vi "climb mode.vi"(4 "i":i32=1508, 6 "Joystick 2":T1, 7 "Arm Angle":dbl=0.38043151000000003, 8 "engage climb":bool, 9 "Button 1":bool, 10 "Slide":dbl(slide)=1.0 scale=0.0..1.0, 11 "Joystick 1 Axes":T2={"Axis 1 (x)"=0.047244094488188976, "Axis 2 (y)"=-0.047244094488188976, "Axis 3 (throttle)"=-1.0, "Axis 4"=0.0, "Axis 5"=0.0, "Axis 6"=0.0}) -> ()   [LabVIEW 2012]
uses:
  <vilib>/Rock Robotics/WPI/Solenoid/WPI_SolenoidValue.ctl
  <vilib>/Rock Robotics/WPI/Joystick/WPI_JoystickGetSetRefNum.vi
  <vilib>/Rock Robotics/WPI/Solenoid/WPI_SolenoidSetEnum.vi
panel:
  out "Arm Motor Output":dbl
  out "Down Range":dbl=0.6
  out "Up Range":dbl=4.1
  out "right f":i32=11868
  out "left f":i32=11868
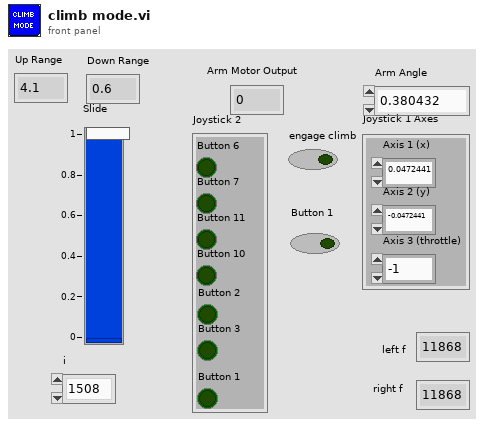
[diagram p1: front panel]
types:
  T1 = cluster{"Button 6":bool, "Button 7":bool, "Button 11":bool, "Button 10":bool, "Button 2":bool, "Button 3":bool, "Button 1":bool}
  T2 = cluster{"Axis 1 (x)":dbl, "Axis 2 (y)":dbl, "Axis 3 (throttle)":dbl, "Axis 4":dbl, "Axis 5":dbl, "Axis 6":dbl}
  T3 = typedef "WPI_SolenoidValue.ctl" = enum16{"Off", "On", "Forward", "Reverse"}
  T4 = typedef "WPI_JoystickDevRef.ctl" = cluster{"Device":T5}
  T5 = typedef "WPI_JoystickDeviceEnum.ctl" = enum16{"USB 1", "USB 2", "USB 3", "USB 4", "Kinect 1", "Kinect 2"}
  T6 = typedef "WPI_JoystickButtonState.ctl" = cluster{"Button 1":bool, "Button 2":bool, "Button 3":bool, "Button 4":bool, "Button 5":bool, "Button 6":bool, "Button 7":bool, "Button 8":bool, "Button 9":bool, "Button 10":bool, "Button 11":bool, "Button 12":bool}
  T7 = typedef "WPI_MotorControlDeviceRef.ctl" = cluster{"DeviceStatus":errorcluster, "Type":enum16{"PWM", "CAN"}, "PWM":cluster{"Digital Module":T8, "PWM Channel":T9, "DeadBand":T10}, "CAN":cluster{"Device Number":u8, "Control Mode":T11, "Semaphore":T12, "Max Vout":dbl}, "Invert":bool, "TransformRef":T13, "InvTransformRef":T13}
  T8 = typedef "FPGA_TypedefDigitalModule.ctl" = enum16{"Digital Module 1", "Digital Module 2"}
  T9 = typedef "FPGA_DIOPWMChannel.ctl" = enum8{"PWM 1", "PWM 2", "PWM 3", "PWM 4", "PWM 5", "PWM 6", "PWM 7", "PWM 8", "PWM 9", "PWM 10", "Invalid"}
  T10 = typedef "WPI_PWMDeadband.ctl" = cluster{"Name":string, "maxPositivePwm":i32, "minPositivePwm":i32, "centerPwm":i32, "maxNegativePwm":i32, "minNegativePwm":i32, "angularRange":u16}
  T11 = typedef "WPI_CANJaguar_ControlMode.ctl" = enum8{"Percent VBus", "Current", "Speed", "Position", "Voltage"}
  T12 = typedef "Semaphore RefNum" = refnum<k1>
  T13 = typedef "WPI_PWMTransform_ConPane.ctl" = refnum<vi>
  T14 = typedef "WPI_SolenoidDevRef.ctl" = cluster{"DevStatus":errorcluster, "Solenoid Module":T15, "Forward Solenoid Channel":T16, "Reverse Solenoid Channel":T16}
  T15 = typedef "FPGA_TypedefSolenoidModule.ctl" = enum16{"Solenoid Module 1", "Solenoid Module 2"}
  T16 = typedef "WPI_SolenoidChannel.ctl" = enum8{"Solenoid 1", "Solenoid 2", "Solenoid 3", "Solenoid 4", "Solenoid 5", "Solenoid 6", "Solenoid 7", "Solenoid 8", "Invalid"}
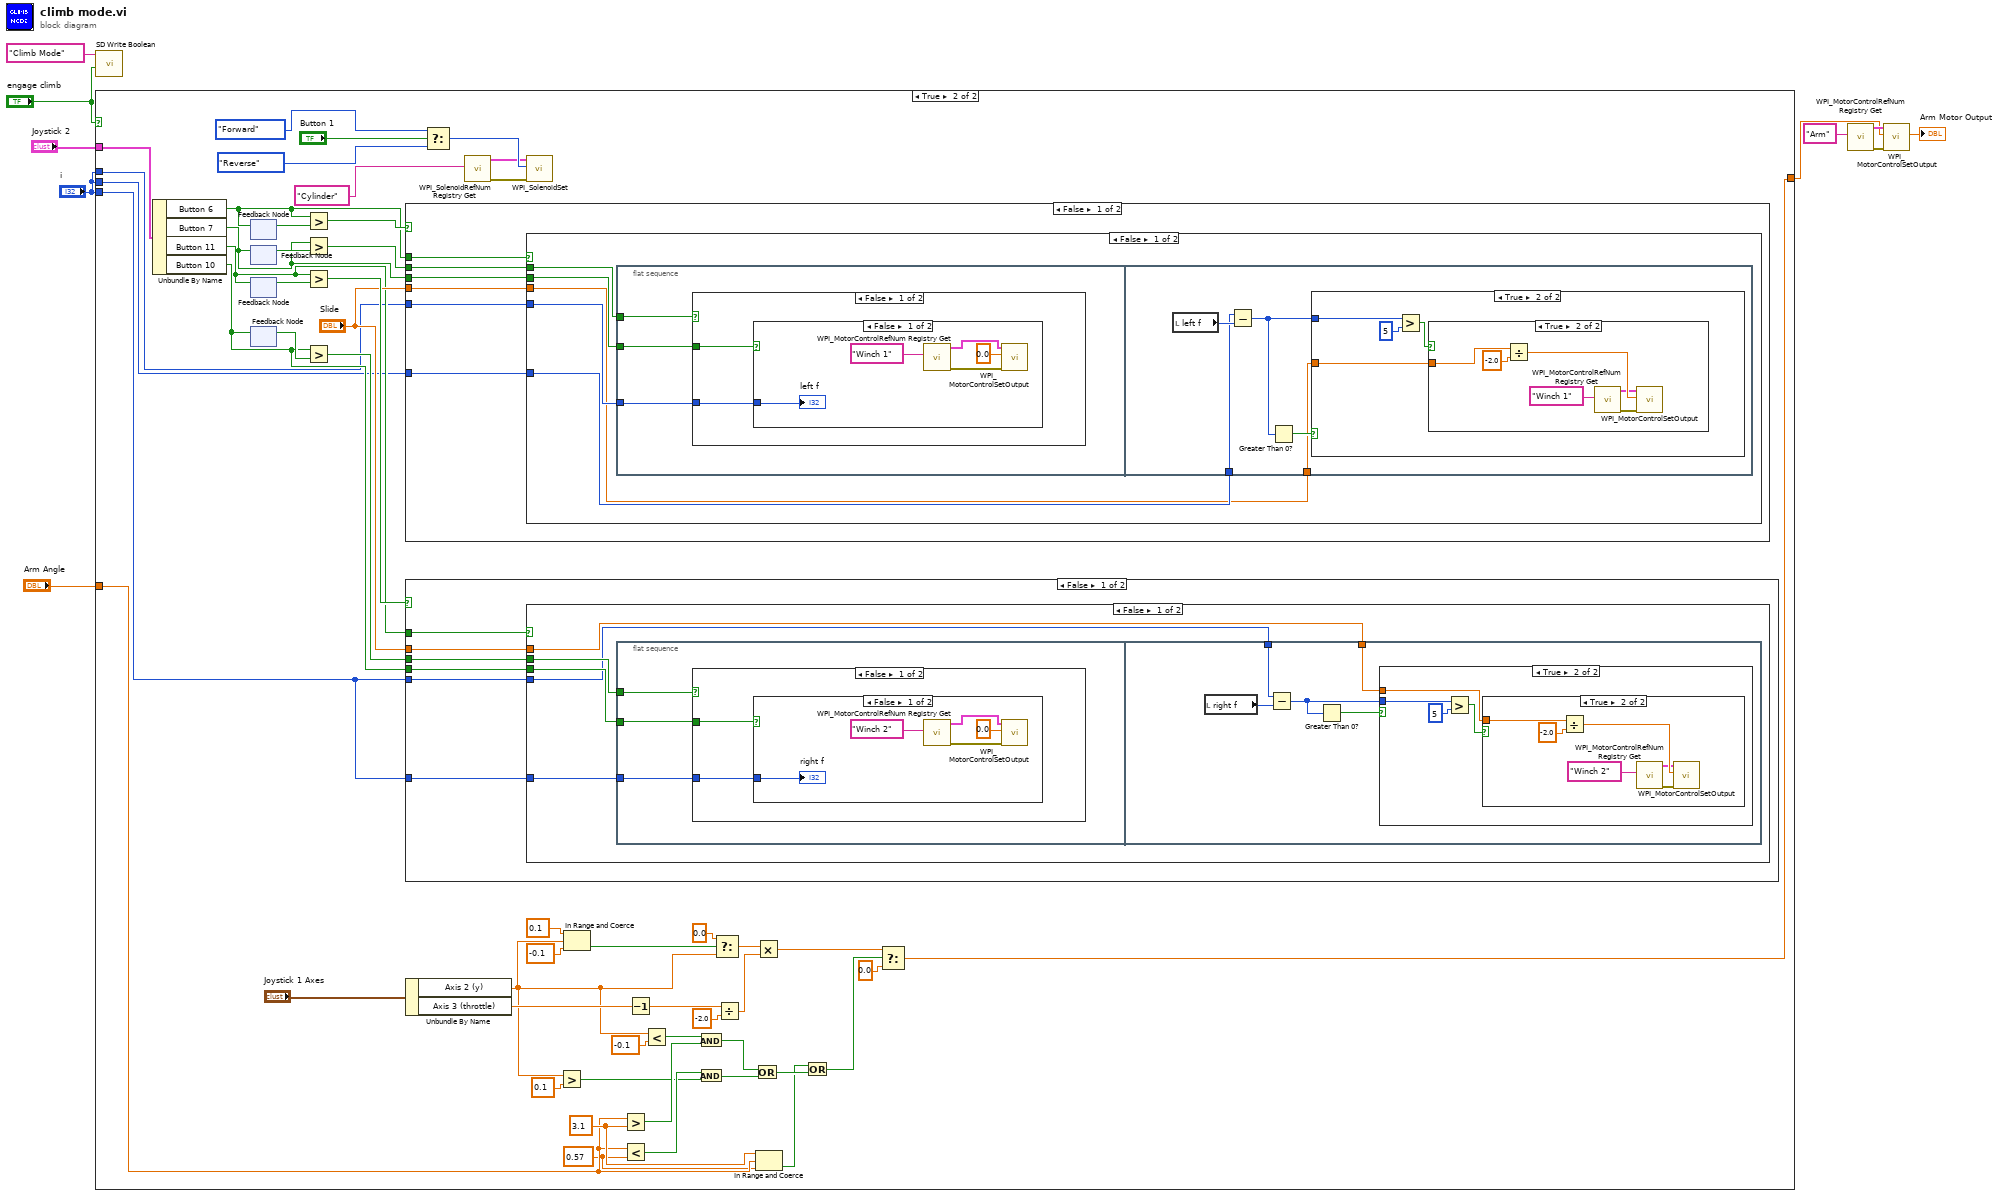
[diagram p0: block diagram]
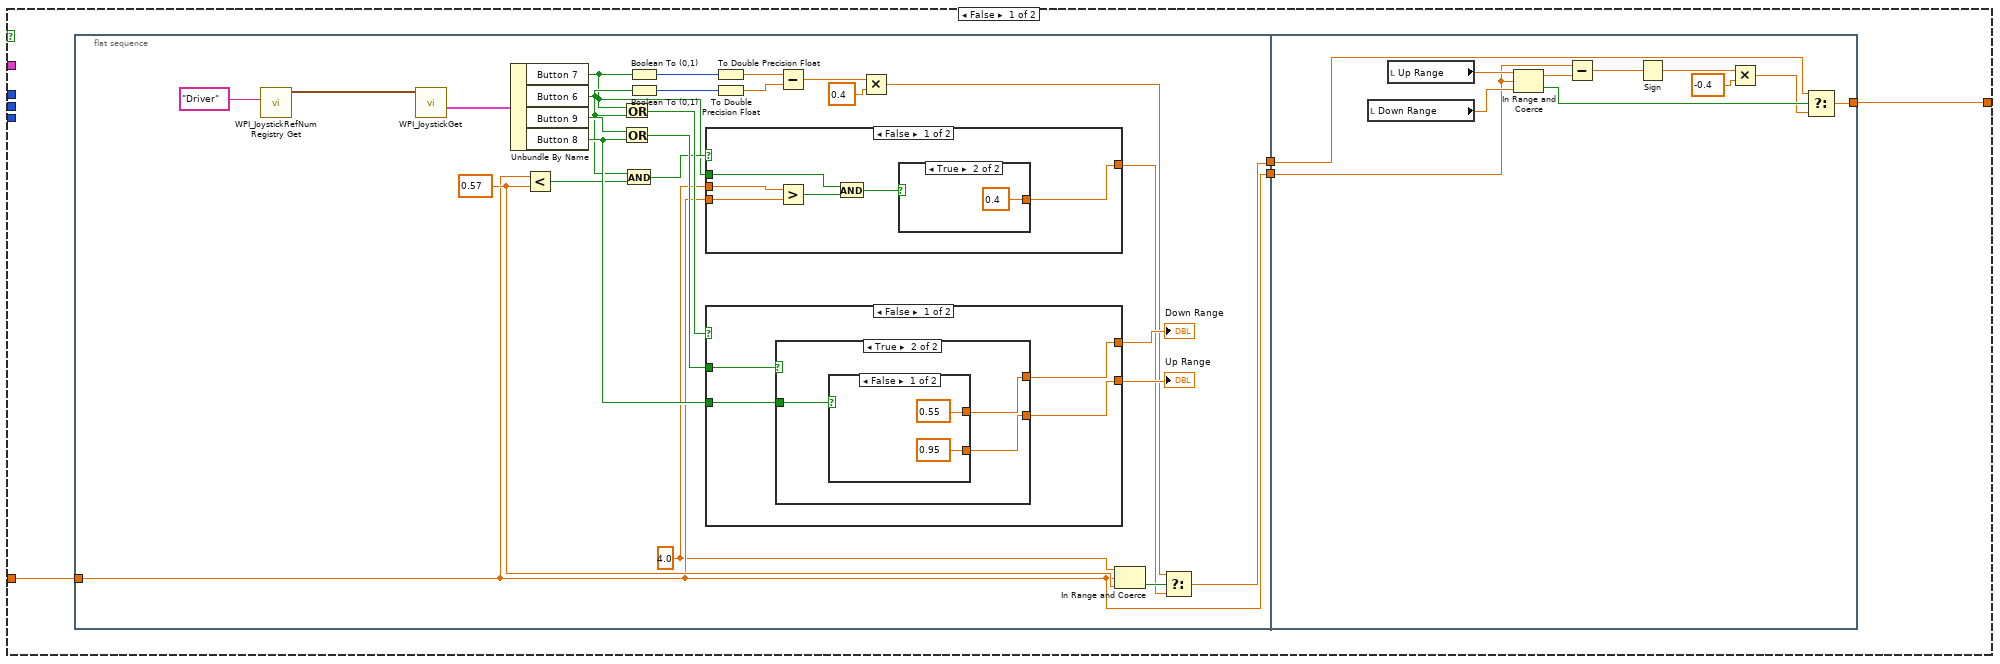
[diagram p2: hidden frame]
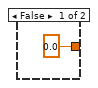
[diagram p3: hidden frame]
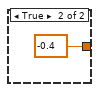
[diagram p4: hidden frame]
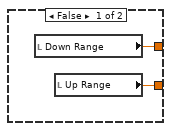
[diagram p5: hidden frame]
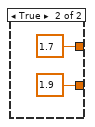
[diagram p6: hidden frame]
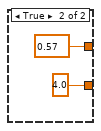
[diagram p7: hidden frame]
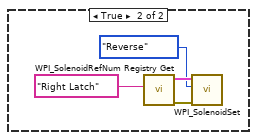
[diagram p8: hidden frame]
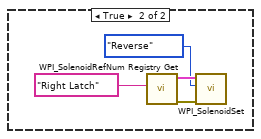
[diagram p9: hidden frame]
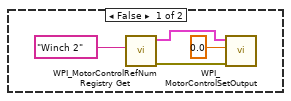
[diagram p10: hidden frame]
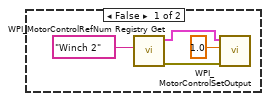
[diagram p11: hidden frame]
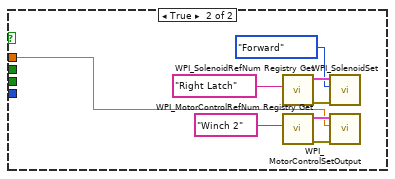
[diagram p12: hidden frame]
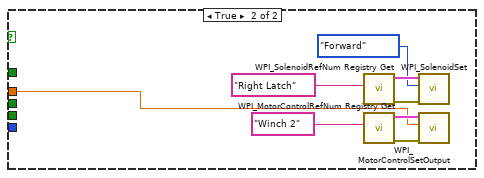
[diagram p13: hidden frame]
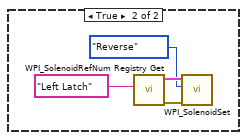
[diagram p14: hidden frame]
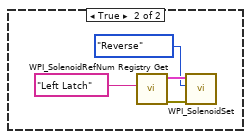
[diagram p15: hidden frame]
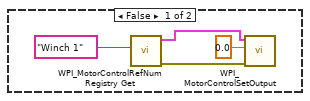
[diagram p16: hidden frame]
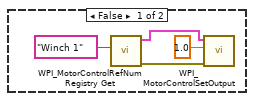
[diagram p17: hidden frame]
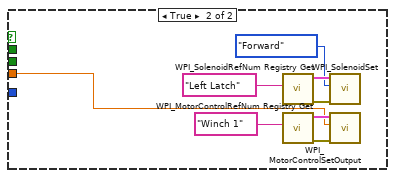
[diagram p18: hidden frame]
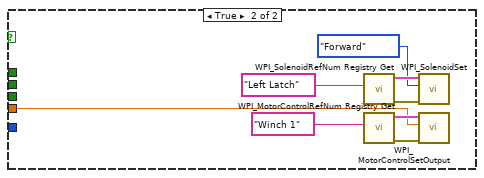
[diagram p19: hidden frame]
diagram:
  n1 = call <vilib>:"SD Write Boolean.vi"("Boolean"="engage climb", "Name"="Climb Mode") -> ()  [unwired: 8 in, 2 out]
  n2 = case shown="True" "engage climb" {
    tunnel: "Joystick 2" -> [_ w119]
    tunnel: "i" -> [_ w105]
    tunnel: "i" -> [_ w104]
    tunnel: "i" -> [_ w103]
    tunnel: "Arm Angle" -> [w14 w86]
    tunnel: [w11 w92] -> w2
    frame False {
      n3 = flat-sequence {
        tunnel: w14 -> [w16]
        tunnel: [w23] -> w13
        tunnel: [w16] -> w12
        tunnel: w13 -> [w66]
        tunnel: w12 -> [w71]
        tunnel: [w65] -> w11
        frame #0 {
          w22 = 0.57 ("lower limit")
          w15 = 4.0 ("upper limit")
          n4 = call <vilib>:"WPI_JoystickRefNum Registry Get.vi"("refnum name"="Driver") -> ("JoystickDevRef"=w40:T4)  [unwired: 9 in, 1 out]
          n5 = call <vilib>:"WPI_JoystickGet.vi"("JoystickDevRef"=w40) -> ("Buttons"=w38:T6)  [unwired: 4 in, 2 out]
          n6 = Unbundle By Name(w38) -> ("Button 7"=w17:bool, "Button 6"=w18:bool, "Button 9"=w29:bool, "Button 8"=w25:bool)
          n7 = Less?(x=w16, y=w22) -> (x < y?=w20:bool)
          n8 = Or(x=w17, y=w18) -> (x .or. y?=w28:bool)
          n9 = Or(x=w29, y=w25) -> (x .or. y?=w30:bool)
          n10 = And(x=w18, y=w20) -> (x .and. y?=w19:bool)
          n11 = Boolean To (0,1)(Boolean=w17) -> (0, 1=w37:i16)
          n12 = Boolean To (0,1)(Boolean=w18) -> (0, 1=w36:i16)
          n13 = case shown="False" w19 {
            tunnel: [w41 -0.4 ("t")] -> w21
            tunnel: w17 -> [w45 _]
            tunnel: w16 -> [w43 _]
            tunnel: w15 -> [w42 _]
            frame False {
              n14 = Greater?(x=w42, y=w43) -> (0:w44:bool)
              n15 = And(x=w45, y=w44) -> (x .and. y?=w46:bool)
              n16 = case shown="True" w46 {
                tunnel: [0.0 0.4] -> w41
                frame False {
                }
                frame True {
                }
              }
            }
            frame True {
            }
          }
          n17 = case shown="False" w28 {
            tunnel: w30 -> [w53 _]
            tunnel: [w52 4.0] -> w27
            tunnel: [w51 0.57] -> w26
            tunnel: w25 -> [w50 _]
            frame False {
              n18 = case shown="True" w53 {
                tunnel: [w55 w56] -> w52
                tunnel: [w54 w57] -> w51
                tunnel: w50 -> [_ w58]
                frame False {
                  n19 = local read "Down Range"() -> (w54:dbl)
                  n20 = local read "Up Range"() -> (w55:dbl)
                }
                frame True {
                  n21 = case shown="False" w58 {
                    tunnel: [0.55 1.7] -> w57
                    tunnel: [0.95 1.9] -> w56
                    frame False {
                    }
                    frame True {
                    }
                  }
                }
              }
            }
            frame True {
            }
          }
          "Up Range" <- w27
          "Down Range" <- w26
          n22 = To Double Precision Float(number=w37) -> (double precision float=w35:dbl)
          n23 = To Double Precision Float(number=w36) -> (double precision float=w34:dbl)
          n24 = Subtract(x=w35, y=w34) -> (x-y=w32:dbl)
          n25 = Multiply(x=w32, y=0.4) -> (x*y=w24:dbl)
          n26 = In Range and Coerce(upper limit=w15, x=w16, lower limit=w22) -> (In Range?=w31:bool)  [unwired: 1 out]
          n27 = Select(t=w24, s=w31, f=w21) -> (s? t:f=w23:dbl)
        }
        frame #1 {
          n28 = local read "Down Range"() -> (w75:dbl)
          n29 = local read "Up Range"() -> (w74:dbl)
          n30 = In Range and Coerce(upper limit=w74, x=w71, lower limit=w75) -> (coerced(x)=w72:dbl, In Range?=w73:bool)
          n31 = Subtract(x=w71, y=w72) -> (x-y=w70:dbl)
          n32 = Sign(1:w70) -> (0:w69:dbl)
          n33 = Multiply(x=w69, y=-0.4) -> (x*y=w67:dbl)
          n34 = Select(t=w66, s=w73, f=w67) -> (s? t:f=w65:dbl)
        }
      }
    }
    frame True {
      w85 = 0.57 ("lower limit")
      w87 = 3.1 ("upper limit")
      n35 = Unbundle By Name(w119) -> ("Button 6"=w109:bool, "Button 7"=w108:bool, "Button 11"=w107:bool, "Button 10"=w106:bool)
      n36 = feedback-in #1(w109) -> ()
      n37 = feedback #1() -> (w118:bool)  [unwired: 1 in]
      n38 = feedback #2() -> (w117:bool)  [unwired: 1 in]
      n39 = feedback-in #2(w108) -> ()
      n40 = feedback #3() -> (w114:bool)  [unwired: 1 in]
      n41 = feedback-in #3(w107) -> ()
      n42 = feedback #4() -> (w113:bool)  [unwired: 1 in]
      n43 = feedback-in #4(w106) -> ()
      n44 = Greater?(x=w109, y=w118) -> (0:w116:bool)
      n45 = Greater?(x=w108, y=w117) -> (0:w115:bool)
      n46 = Greater?(x=w107, y=w114) -> (0:w112:bool)
      n47 = Greater?(x=w106, y=w113) -> (0:w111:bool)
      n48 = case shown="False" w116 {
        tunnel: "Slide" -> [w200 w256]
        tunnel: w109 -> [w201 _]
        tunnel: w115 -> [w199 _]
        tunnel: w108 -> [w198 _]
        tunnel: w105 -> [w197 _]
        tunnel: w104 -> [w196 _]
        frame False {
          n49 = case shown="False" w201 {
            tunnel: w200 -> [w202 w252]
            tunnel: w198 -> [w206 _]
            tunnel: w199 -> [w205 _]
            tunnel: w197 -> [w204 _]
            tunnel: w196 -> [w203 _]
            frame False {
              n50 = flat-sequence {
                tunnel: w206 -> [w209]
                tunnel: w205 -> [w208]
                tunnel: w204 -> [w207]
                tunnel: w203 -> [w226]
                tunnel: w202 -> [w225]
                frame #0 {
                  n51 = case shown="False" w208 {
                    tunnel: w209 -> [w211 _]
                    tunnel: w207 -> [w210 _]
                    frame False {
                      n52 = case shown="False" w211 {
                        tunnel: w210 -> [w216 _]
                        frame False {
                          n53 = call <vilib>:"WPI_MotorControlRefNum Registry Get.vi"("refnum name"="Winch 1") -> ("error out"=w215:errorcluster, "MotorControlDevRef"=w213:T7)  [unwired: 9 in]
                          n54 = call <vilib>:"WPI_MotorControlSetOutput.vi"("error in (no error)"=w215, "Output"=0.0, "MotorControlDevRef"=w213) -> ()  [unwired: 6 in, 3 out]
                          "left f" <- w216
                        }
                        frame True {
                          n55 = call <vilib>:"WPI_SolenoidRefNum Registry Get.vi"("refnum name"="Left Latch") -> ("error out"=w220:errorcluster, "SolenoidDevRef"=w218:T14)  [unwired: 9 in]
                          n56 = call-poly <vilib>:"WPI_SolenoidSet.vi"("error in (no error)"=w220, "Value"=WPI_SolenoidValue."Reverse", "SolenoidDevRef"=w218) -> ()  [unwired: 7 in, 2 out]
                        }
                      }
                    }
                    frame True {
                      n57 = call <vilib>:"WPI_SolenoidRefNum Registry Get.vi"("refnum name"="Left Latch") -> ("error out"=w224:errorcluster, "SolenoidDevRef"=w222:T14)  [unwired: 9 in]
                      n58 = call-poly <vilib>:"WPI_SolenoidSet.vi"("error in (no error)"=w224, "Value"=WPI_SolenoidValue."Reverse", "SolenoidDevRef"=w222) -> ()  [unwired: 7 in, 2 out]
                    }
                  }
                }
                frame #1 {
                  n59 = local read "left f"() -> (w228:i32)
                  n60 = Subtract(x=w226, y=w228) -> (x-y=w229:i32)
                  n61 = Greater Than 0?(x=w229) -> (x > 0?=w227:bool)
                  n62 = case shown="True" w227 {
                    tunnel: w229 -> [_ w235]
                    tunnel: w225 -> [_ w234]
                    frame False {
                      n63 = call <vilib>:"WPI_MotorControlRefNum Registry Get.vi"("refnum name"="Winch 1") -> ("error out"=w233:errorcluster, "MotorControlDevRef"=w231:T7)  [unwired: 9 in]
                      n64 = call <vilib>:"WPI_MotorControlSetOutput.vi"("error in (no error)"=w233, "Output"=0.0, "MotorControlDevRef"=w231) -> ()  [unwired: 6 in, 3 out]
                    }
                    frame True {
                      n65 = Greater?(x=w235, y=5) -> (0:w237:bool)
                      n66 = case shown="True" w237 {
                        tunnel: w234 -> [_ w242]
                        frame False {
                          n67 = call <vilib>:"WPI_MotorControlRefNum Registry Get.vi"("refnum name"="Winch 1") -> ("error out"=w241:errorcluster, "MotorControlDevRef"=w239:T7)  [unwired: 9 in]
                          n68 = call <vilib>:"WPI_MotorControlSetOutput.vi"("error in (no error)"=w241, "Output"=1.0, "MotorControlDevRef"=w239) -> ()  [unwired: 6 in, 3 out]
                        }
                        frame True {
                          n69 = Divide(x=w242, y=-2.0) -> (x/y=w247:dbl)
                          n70 = call <vilib>:"WPI_MotorControlRefNum Registry Get.vi"("refnum name"="Winch 1") -> ("error out"=w246:errorcluster, "MotorControlDevRef"=w244:T7)  [unwired: 9 in]
                          n71 = call <vilib>:"WPI_MotorControlSetOutput.vi"("error in (no error)"=w246, "Output"=w247, "MotorControlDevRef"=w244) -> ()  [unwired: 6 in, 3 out]
                        }
                      }
                    }
                  }
                }
              }
            }
            frame True {
              n72 = call <vilib>:"WPI_SolenoidRefNum Registry Get.vi"("refnum name"="Left Latch") -> ("error out"=w251:errorcluster, "SolenoidDevRef"=w249:T14)  [unwired: 9 in]
              n73 = call <vilib>:"WPI_MotorControlRefNum Registry Get.vi"("refnum name"="Winch 1") -> ("error out"=w255:errorcluster, "MotorControlDevRef"=w253:T7)  [unwired: 9 in]
              n74 = call-poly <vilib>:"WPI_SolenoidSet.vi"("error in (no error)"=w251, "Value"=WPI_SolenoidValue."Forward", "SolenoidDevRef"=w249) -> ()  [unwired: 7 in, 2 out]
              n75 = call <vilib>:"WPI_MotorControlSetOutput.vi"("error in (no error)"=w255, "Output"=w252, "MotorControlDevRef"=w253) -> ()  [unwired: 6 in, 3 out]
            }
          }
        }
        frame True {
          n76 = call <vilib>:"WPI_SolenoidRefNum Registry Get.vi"("refnum name"="Left Latch") -> ("error out"=w263:errorcluster, "SolenoidDevRef"=w261:T14)  [unwired: 9 in]
          n77 = call <vilib>:"WPI_MotorControlRefNum Registry Get.vi"("refnum name"="Winch 1") -> ("error out"=w259:errorcluster, "MotorControlDevRef"=w257:T7)  [unwired: 9 in]
          n78 = call-poly <vilib>:"WPI_SolenoidSet.vi"("error in (no error)"=w263, "Value"=WPI_SolenoidValue."Forward", "SolenoidDevRef"=w261) -> ()  [unwired: 7 in, 2 out]
          n79 = call <vilib>:"WPI_MotorControlSetOutput.vi"("error in (no error)"=w259, "Output"=w256, "MotorControlDevRef"=w257) -> ()  [unwired: 6 in, 3 out]
        }
      }
      n80 = case shown="False" w112 {
        tunnel: "Slide" -> [w132 w188]
        tunnel: w107 -> [w133 _]
        tunnel: w111 -> [w131 _]
        tunnel: w106 -> [w130 _]
        tunnel: w103 -> [w129 _]
        tunnel: w103 -> [w128 _]
        frame False {
          n81 = case shown="False" w133 {
            tunnel: w132 -> [w134 w184]
            tunnel: w130 -> [w138 _]
            tunnel: w131 -> [w137 _]
            tunnel: w129 -> [w135 _]
            tunnel: w128 -> [w136 _]
            frame False {
              n82 = flat-sequence {
                tunnel: w138 -> [w141]
                tunnel: w137 -> [w140]
                tunnel: w136 -> [w139]
                tunnel: w135 -> [w158]
                tunnel: w134 -> [w157]
                frame #0 {
                  n83 = case shown="False" w140 {
                    tunnel: w141 -> [w143 _]
                    tunnel: w139 -> [w142 _]
                    frame False {
                      n84 = case shown="False" w143 {
                        tunnel: w142 -> [w148 _]
                        frame False {
                          n85 = call <vilib>:"WPI_MotorControlRefNum Registry Get.vi"("refnum name"="Winch 2") -> ("error out"=w147:errorcluster, "MotorControlDevRef"=w145:T7)  [unwired: 9 in]
                          n86 = call <vilib>:"WPI_MotorControlSetOutput.vi"("error in (no error)"=w147, "Output"=0.0, "MotorControlDevRef"=w145) -> ()  [unwired: 6 in, 3 out]
                          "right f" <- w148
                        }
                        frame True {
                          n87 = call <vilib>:"WPI_SolenoidRefNum Registry Get.vi"("refnum name"="Right Latch") -> ("error out"=w152:errorcluster, "SolenoidDevRef"=w150:T14)  [unwired: 9 in]
                          n88 = call-poly <vilib>:"WPI_SolenoidSet.vi"("error in (no error)"=w152, "Value"=WPI_SolenoidValue."Reverse", "SolenoidDevRef"=w150) -> ()  [unwired: 7 in, 2 out]
                        }
                      }
                    }
                    frame True {
                      n89 = call <vilib>:"WPI_SolenoidRefNum Registry Get.vi"("refnum name"="Right Latch") -> ("error out"=w156:errorcluster, "SolenoidDevRef"=w154:T14)  [unwired: 9 in]
                      n90 = call-poly <vilib>:"WPI_SolenoidSet.vi"("error in (no error)"=w156, "Value"=WPI_SolenoidValue."Reverse", "SolenoidDevRef"=w154) -> ()  [unwired: 7 in, 2 out]
                    }
                  }
                }
                frame #1 {
                  n91 = local read "right f"() -> (w160:i32)
                  n92 = Subtract(x=w158, y=w160) -> (x-y=w161:i32)
                  n93 = Greater Than 0?(x=w161) -> (x > 0?=w159:bool)
                  n94 = case shown="True" w159 {
                    tunnel: w161 -> [_ w167]
                    tunnel: w157 -> [_ w166]
                    frame False {
                      n95 = call <vilib>:"WPI_MotorControlRefNum Registry Get.vi"("refnum name"="Winch 2") -> ("error out"=w165:errorcluster, "MotorControlDevRef"=w163:T7)  [unwired: 9 in]
                      n96 = call <vilib>:"WPI_MotorControlSetOutput.vi"("error in (no error)"=w165, "Output"=0.0, "MotorControlDevRef"=w163) -> ()  [unwired: 6 in, 3 out]
                    }
                    frame True {
                      n97 = Greater?(x=w167, y=5) -> (0:w169:bool)
                      n98 = case shown="True" w169 {
                        tunnel: w166 -> [_ w174]
                        frame False {
                          n99 = call <vilib>:"WPI_MotorControlRefNum Registry Get.vi"("refnum name"="Winch 2") -> ("error out"=w173:errorcluster, "MotorControlDevRef"=w171:T7)  [unwired: 9 in]
                          n100 = call <vilib>:"WPI_MotorControlSetOutput.vi"("error in (no error)"=w173, "Output"=1.0, "MotorControlDevRef"=w171) -> ()  [unwired: 6 in, 3 out]
                        }
                        frame True {
                          n101 = Divide(x=w174, y=-2.0) -> (x/y=w179:dbl)
                          n102 = call <vilib>:"WPI_MotorControlRefNum Registry Get.vi"("refnum name"="Winch 2") -> ("error out"=w178:errorcluster, "MotorControlDevRef"=w176:T7)  [unwired: 9 in]
                          n103 = call <vilib>:"WPI_MotorControlSetOutput.vi"("error in (no error)"=w178, "Output"=w179, "MotorControlDevRef"=w176) -> ()  [unwired: 6 in, 3 out]
                        }
                      }
                    }
                  }
                }
              }
            }
            frame True {
              n104 = call <vilib>:"WPI_SolenoidRefNum Registry Get.vi"("refnum name"="Right Latch") -> ("error out"=w183:errorcluster, "SolenoidDevRef"=w181:T14)  [unwired: 9 in]
              n105 = call <vilib>:"WPI_MotorControlRefNum Registry Get.vi"("refnum name"="Winch 2") -> ("error out"=w187:errorcluster, "MotorControlDevRef"=w185:T7)  [unwired: 9 in]
              n106 = call-poly <vilib>:"WPI_SolenoidSet.vi"("error in (no error)"=w183, "Value"=WPI_SolenoidValue."Forward", "SolenoidDevRef"=w181) -> ()  [unwired: 7 in, 2 out]
              n107 = call <vilib>:"WPI_MotorControlSetOutput.vi"("error in (no error)"=w187, "Output"=w184, "MotorControlDevRef"=w185) -> ()  [unwired: 6 in, 3 out]
            }
          }
        }
        frame True {
          n108 = call <vilib>:"WPI_SolenoidRefNum Registry Get.vi"("refnum name"="Right Latch") -> ("error out"=w195:errorcluster, "SolenoidDevRef"=w193:T14)  [unwired: 9 in]
          n109 = call <vilib>:"WPI_MotorControlRefNum Registry Get.vi"("refnum name"="Winch 2") -> ("error out"=w191:errorcluster, "MotorControlDevRef"=w189:T7)  [unwired: 9 in]
          n110 = call-poly <vilib>:"WPI_SolenoidSet.vi"("error in (no error)"=w195, "Value"=WPI_SolenoidValue."Forward", "SolenoidDevRef"=w193) -> ()  [unwired: 7 in, 2 out]
          n111 = call <vilib>:"WPI_MotorControlSetOutput.vi"("error in (no error)"=w191, "Output"=w188, "MotorControlDevRef"=w189) -> ()  [unwired: 6 in, 3 out]
        }
      }
      n112 = Unbundle By Name("Joystick 1 Axes") -> ("Axis 2 (y)"=w76:dbl, "Axis 3 (throttle)"=w82:dbl)
      n113 = Select(t=WPI_SolenoidValue."Forward", s="Button 1", f=WPI_SolenoidValue."Reverse" ("Value")) -> (s? t:f=w124:T3)
      n114 = call <vilib>:"WPI_SolenoidRefNum Registry Get.vi"("refnum name"="Cylinder") -> ("error out"=w120:errorcluster, "SolenoidDevRef"=w123:T14)  [unwired: 9 in]
      n115 = call-poly <vilib>:"WPI_SolenoidSet.vi"("error in (no error)"=w120, "Value"=w124, "SolenoidDevRef"=w123) -> ()  [unwired: 7 in, 2 out]
      n116 = Greater?(x=w76, y=0.1) -> (0:w80:bool)
      n117 = In Range and Coerce(upper limit=0.1, x=w76, lower limit=-0.1) -> (In Range?=w95:bool)  [unwired: 1 out]
      n118 = Greater?(x=w86, y=w87) -> (0:w91:bool)
      n119 = Less?(x=w86, y=w85) -> (x < y?=w89:bool)
      n120 = Decrement(x=w82) -> (x-1=w101:dbl)
      n121 = Less?(x=w76, y=-0.1) -> (x < y?=w83:bool)
      n122 = And(x=w83, y=w91) -> (x .and. y?=w90:bool)
      n123 = And(x=w89, y=w80) -> (x .and. y?=w88:bool)
      n124 = Select(t=0.0, s=w95, f=w76) -> (s? t:f=w93:dbl)
      n125 = Divide(x=w101, y=-2.0) -> (x/y=w99:dbl)
      n126 = Or(x=w90, y=w88) -> (x .or. y?=w79:bool)
      n127 = Multiply(x=w93, y=w99) -> (x*y=w98:dbl)
      n128 = In Range and Coerce(upper limit=w87, x=w86, lower limit=w85) -> (In Range?=w78:bool)  [unwired: 1 out]
      n129 = Or(x=w78, y=w79) -> (x .or. y?=w77:bool)
      n130 = Select(t=w98, s=w77, f=0.0) -> (s? t:f=w92:dbl)
    }
  }
  n131 = call <vilib>:"WPI_MotorControlRefNum Registry Get.vi"("refnum name"="Arm") -> ("error out"=w4:errorcluster, "MotorControlDevRef"=w3:T7)  [unwired: 9 in]
  n132 = call <vilib>:"WPI_MotorControlSetOutput.vi"("error in (no error)"=w4, "Output"=w2, "MotorControlDevRef"=w3) -> ("Motor Output"=→"Arm Motor Output":dbl)  [unwired: 6 in, 2 out]
